vi "Application Version.vi"() -> (3 "Application Version":string)   [LabVIEW 2018]
doc: "Get the version information for the built application. Returns \"Development\" when running from LabVIEW."
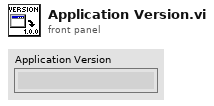
[diagram p1: front panel]
types:
  T1 = enum32{"invalid app kind", "Development System", "Run Time System", "Student Edition", "Embedded LabVIEW", "Evaluation", "Custom"}
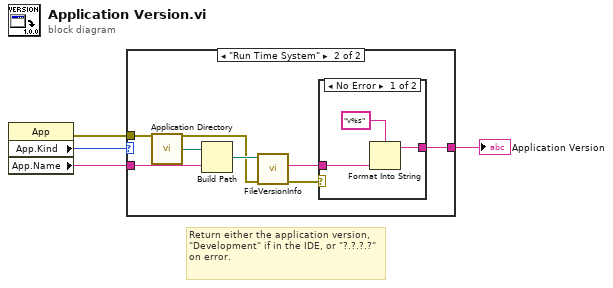
[diagram p0: block diagram]
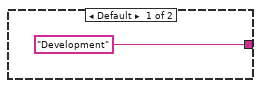
[diagram p2: hidden frame]
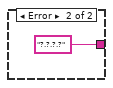
[diagram p3: hidden frame]
diagram:
  # "Return either the application version, \"Development\" if in the IDE, or \"?.?.?.?\" on error."
  n1 = property class="App"() -> (error out=w1:errorcluster, "App.Kind"=w2:T1, "App.Name"=w3:string)  [unwired: 2 in, 1 out]
  n2 = case shown="\"Run Time System\"" w2 {
    tunnel: ["Development" ("File Version Info") w8] -> w4
    tunnel: w3 -> [_ w11]
    tunnel: w1 -> [_ w7]
    frame Default {
    }
    frame "Run Time System" {
      n3 = call <vilib>:"Application Directory.vi"() -> ("Application Directory"=w12:path)
      n4 = Build Path(base path=w12, name or relative path=w11) -> (appended path=w10:path)
      n5 = call <vilib>:"FileVersionInfo.vi"("error in (no error)"=w7, "Application Path in"=w10) -> ("error out"=w6:errorcluster, "File Version Info"=w9:string)  [unwired: 6 in, 2 out]
      n6 = case shown="No Error" w6 {
        tunnel: w9 -> [w14 _]
        tunnel: [w13 "?.?.?.?"] -> w8
        frame No Error {
          n7 = Format Into String(format string="v%s", w14) -> (resulting string=w13:string)  [unwired: 2 in, 1 out]
        }
        frame Error {
        }
      }
    }
  }
  "Application Version" <- w4
